vi "Modify Signal Phase.vi"() -> ()   [LabVIEW 2015]
uses:
  <vilib>/measure/NI_MABase.lvlib
panel:
  in  "Test":bool
  out "Waveform Graph":dbl[][](graph)
  in  "Phase Shift (degree)":dbl
  in  "Input":cdb[](array[numeric])
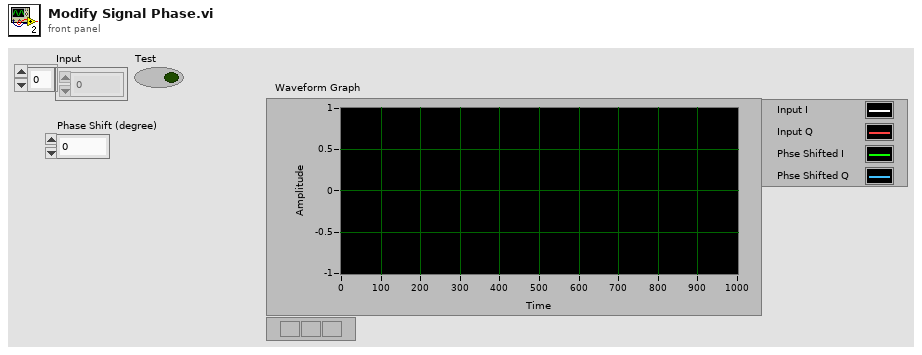
[diagram p1: front panel]
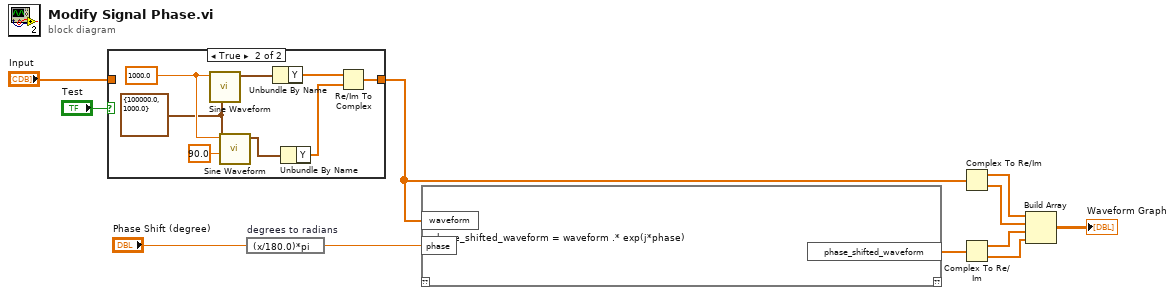
[diagram p0: block diagram]
diagram:
  n1 = case shown="True" "Test" {
    tunnel: [w12 w13] -> w9
    tunnel: "Input" -> [w12 _]
    frame False {
    }
    frame True {
      w17 = cluster{"Fs":dbl, "#s":dbl} {"Fs"=100000.0, "#s"=1000.0} ("sampling info")
      w19 = 1000.0 ("frequency")
      n2 = call <vilib>:"Sine Waveform.vi"("sampling info"=w17, "frequency"=w19) -> ("signal out"=w20:waveform(dbl))  [unwired: 8 in, 1 out]
      n3 = call <vilib>:"Sine Waveform.vi"("sampling info"=w17, "phase"=90.0, "frequency"=w19) -> ("signal out"=w16:waveform(dbl))  [unwired: 7 in, 1 out]
      n4 = Unbundle By Name(w20) -> ("Y"=w15:dbl[])
      n5 = Unbundle By Name(w16) -> ("Y"=w14:dbl[])
      n6 = Re/Im To Complex(1:w14, 2:w15) -> (0:w13:cdb[])
    }
  }
  n7 = expression code="(x/180.0)*pi" "degrees to radians"("Phase Shift (degree)") -> (w10:dbl)
  n8 = mathscript code="phase_shifted_waveform = waveform .* exp(j*phase)"("waveform"=w9, "phase"=w10) -> ("phase_shifted_waveform"=w8:cdb[])  [unwired: 1 in, 1 out]
  n9 = Complex To Re/Im(x + iy=w9) -> (x=w7:dbl[], y=w6:dbl[])
  n10 = Complex To Re/Im(x + iy=w8) -> (x=w5:dbl[], y=w4:dbl[])
  n11 = Build Array(w7, w6, w5, w4) -> (→"Waveform Graph":dbl[][])
